vi "MathOptim-Sigmoid Estimate.vi"(0 "Y":dbl[](array[numeric]), 5 "X":dbl[](array[numeric])) -> (4 "Initial guess":dbl[](array[numeric]))   [LabVIEW 2020]
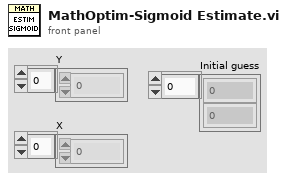
[diagram p1: front panel]
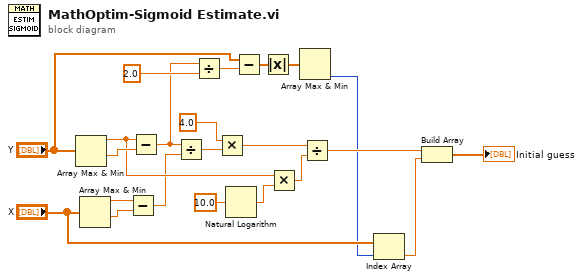
[diagram p0: block diagram]
diagram:
  n1 = Array Max & Min(array="Y") -> (max value=w15:dbl, min value=w19:dbl)  [unwired: 2 out]
  n2 = Array Max & Min(array="X") -> (max value=w21:dbl, min value=w20:dbl)  [unwired: 2 out]
  n3 = Subtract(x=w21, y=w20) -> (x-y=w10:dbl)
  n4 = Subtract(x=w15, y=w19) -> (x-y=w1:dbl)
  n5 = Divide(x=w1, y=w10) -> (x/y=w18:dbl)
  n6 = Divide(x=w1, y=2.0) -> (x/y=w8:dbl)
  n7 = Multiply(x=4.0, y=w18) -> (x*y=w16:dbl)
  n8 = Natural Logarithm(1:10.0 ("x")) -> (0:w13:dbl)
  n9 = Subtract(x="Y", y=w8) -> (x-y=w6:dbl[])
  n10 = Absolute Value(x=w6) -> (abs(x)=w5:dbl[])
  n11 = Multiply(x=w15, y=w13) -> (x*y=w14:dbl)
  n12 = Array Max & Min(array=w5) -> (min index (indices)=w3:i32)  [unwired: 3 out]
  n13 = Divide(x=w16, y=w14) -> (x/y=w11:dbl)
  n14 = Index Array(array="X", index=w3) -> (element=w2:dbl)
  n15 = Build Array(w11, w2) -> (→"Initial guess":dbl[])
